vi "Get VI Name (without extension).vi"() -> (3 "VI Name (without extension)":string)   [LabVIEW 2015, in "Utility.lvlib"]
uses:
  Utility.lvlib
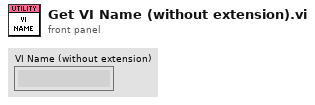
[diagram p1: front panel]
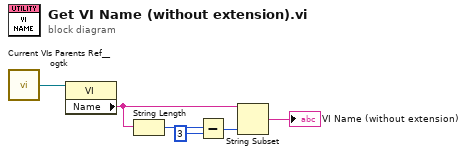
[diagram p0: block diagram]
diagram:
  n1 = call <userlib>:"Current VIs Parents Ref__ogtk.vi"() -> ("Calling VI's Reference"=w6:refnum<vi>)  [unwired: 2 in]
  n2 = property class="VI"(reference=w6) -> ("Name"=w3:string)  [unwired: 1 in, 2 out]
  n3 = String Length(string=w3) -> (length=w5:i32)
  n4 = Subtract(x=w5, y=3) -> (x-y=w2:i32)
  n5 = String Subset(string=w3, length (rest)=w2) -> (substring=→"VI Name (without extension)":string)  [unwired: 1 in]
